vi "TwoPointCaculateAngle-180to+180.vi"(2 "Point2":T1, 4 "Point1":T1) -> (0 "deg( «×)":dbl)   [LabVIEW 2014]
uses:
  Controls/XYZPos.ctl
  <vilib>/vision/NI_Vision_Development_Module.lvlib
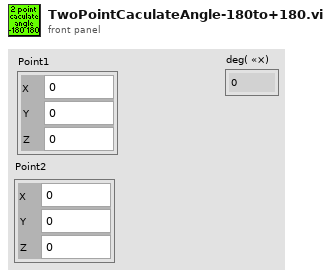
[diagram p1: front panel]
types:
  T1 = typedef "XYZPos.ctl" = cluster{"X":dbl, "Y":dbl, "Z":dbl}
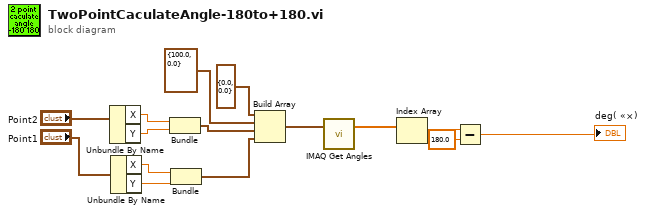
[diagram p0: block diagram]
diagram:
  n1 = Unbundle By Name("Point2") -> ("X"=w5:dbl, "Y"=w6:dbl)
  n2 = Unbundle By Name("Point1") -> ("X"=w3:dbl, "Y"=w2:dbl)
  n3 = Bundle("X"=w5, "Y"=w6) -> (w4:cluster{"X":dbl, "Y":dbl})  [unwired: 1 in]
  n4 = Bundle("X"=w3, "Y"=w2) -> (w1:cluster{"X":dbl, "Y":dbl})  [unwired: 1 in]
  n5 = Build Array(cluster{"X":dbl, "Y":dbl} {"X"=0.0, "Y"=0.0} ("element"), cluster{"X":dbl, "Y":dbl} {"X"=100.0, "Y"=0.0} ("element"), w4, w1) -> (w15:cluster{"X":dbl, "Y":dbl}[])
  n6 = call "IMAQ Get Angles"("Points"=w15) -> ("Angles (deg)"=w14:sgl[])  [unwired: 4 in, 2 out]
  n7 = Index Array(array=w14) -> (element=w11:sgl)  [unwired: 1 in]
  n8 = Subtract(x=w11, y=sgl 180.0) -> (x-y=→"deg( «×)":sgl)
